vi "Write Mfg Serial Number.vi"(8 "error in":errorcluster, 10 "Start Address":u8=171 format="%x", 11 "Serial Number":string) -> (0 "error out":errorcluster)   [LabVIEW 2015]
uses:
  CAN Communication/Gas/Gas.lvclass
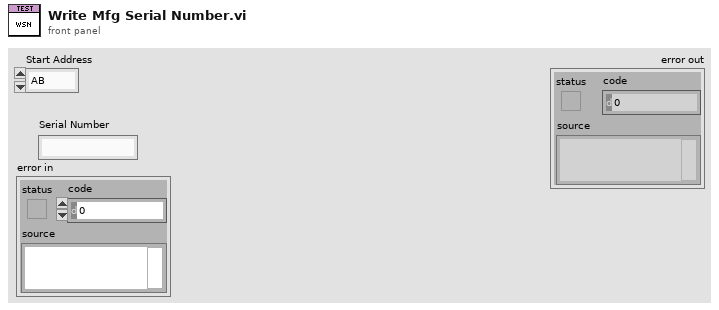
[diagram p1: front panel]
types:
  T1 = typedef "Gas.lvclass/Session Handle.ctl" = refnum<data-value>
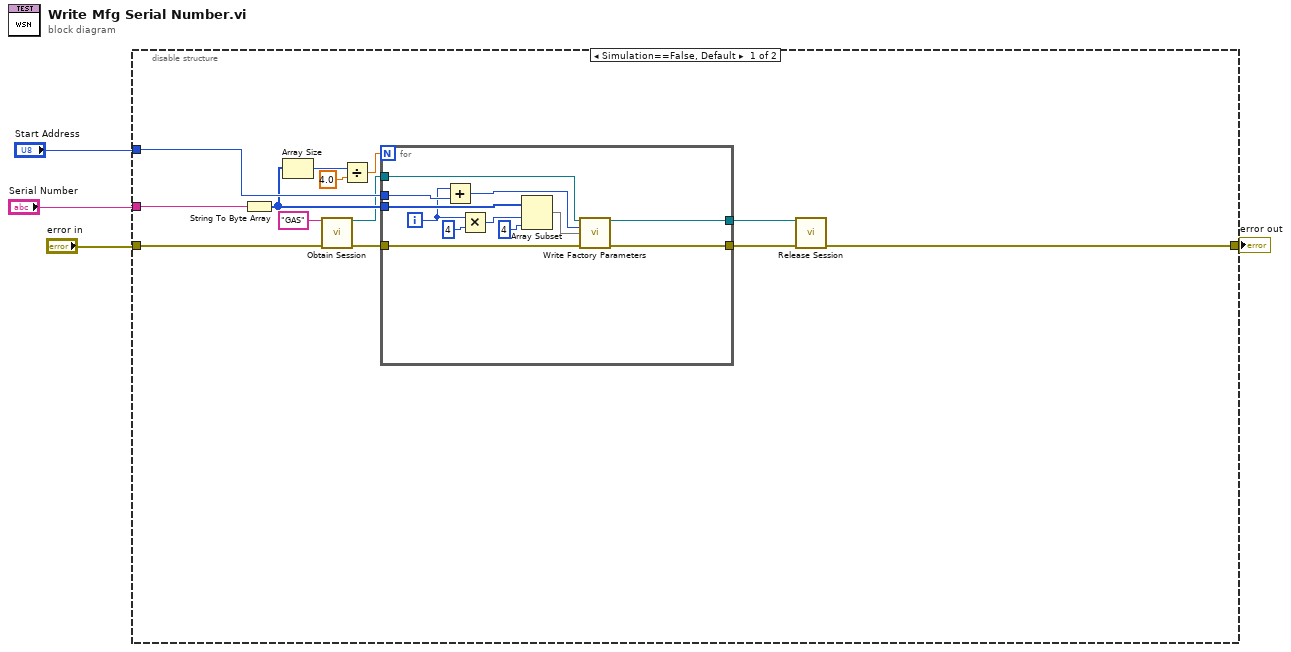
[diagram p0: block diagram]
diagram:
  n1 = disable-structure shown="Simulation==False, Default" {
    disable-tunnel: "error in" -> [w10 w30]
    disable-tunnel: [w5 w30] -> w3
    disable-tunnel: "Serial Number" -> [w16 _]
    disable-tunnel: "Start Address" -> [w17 _]
    frame condition #0 (active) {
      n2 = String To Byte Array(string=w16) -> (unsigned byte array=w13:u8[])
      n3 = Array Size(array=w13) -> (size(s)=w12:i32)
      n4 = call "Obtain Session.vi"("Session  Name ()"="GAS", "error in (no error)"=w10) -> ("Session Handle"=w9:T1, "error out"=w8:errorcluster)  [unwired: 12 in]
      n5 = Divide(x=w12, y=4.0) -> (x/y=w15:dbl)
      n6 = for {
        N: w15 -> [_]
        tunnel: w13 -> [w29]
        tunnel: w17 -> [w24]
        tunnel: w9 -> [w20]
        tunnel: w8 -> [w21]
        tunnel: [w19] -> w7
        tunnel: [w18] -> w6
        i -> [w23]
        n7 = Add(x=w23, y=w24) -> (x+y=w22:i32)
        n8 = Multiply(x=w23, y=4) -> (x*y=w26:i32)
        n9 = Array Subset(array=w29, index=w26, length=4) -> (w25:u8[])
        n10 = call "Write Factory Parameters.vi"("Session Handle in"=w20, "Address"=w22, "Bytes to Write"=w25, "error in (no error)"=w21) -> ("Session Handle out"=w19:T1, "error out"=w18:errorcluster)  [unwired: 10 in]
      }
      n11 = call "Release Session.vi"("Session Handle"=w7, "error in (no error)"=w6) -> ("error out"=w5:errorcluster)  [unwired: 13 in]
    }
    frame condition #1 {
    }
  }
  "error out" <- w3
